vi "VI Tree.vi"   [LabVIEW 2019, in "Agilent 681x Series.lvlib"]
doc: "This is the instrument driver for the Agilent 681x Series. The VI Tree displays all the user-callable VIs of the instrument driver in an organized table."
uses:
  <instrlib>/Agilent 681x Series/Agilent 681x Series.lvlib
  <instrlib>/Agilent 681x Series/Public/Data/Low Level/Fetch Multiple Measurements (Current Data).vi
  <instrlib>/Agilent 681x Series/Public/Data/Read Multiple Measurements (Current Data).vi
  <instrlib>/Agilent 681x Series/Public/Data/Read Single Measurement (Current Harmonics).vi
  <instrlib>/Agilent 681x Series/Public/Data/Low Level/Fetch Single Measurement (Current Harmonics).vi
panel:
  # "(c) 2008-2021 National Instruments Corp.  ALL RIGHTS RESERVED."
  # "SEE DIAGRAM\nFOR VI TREE."
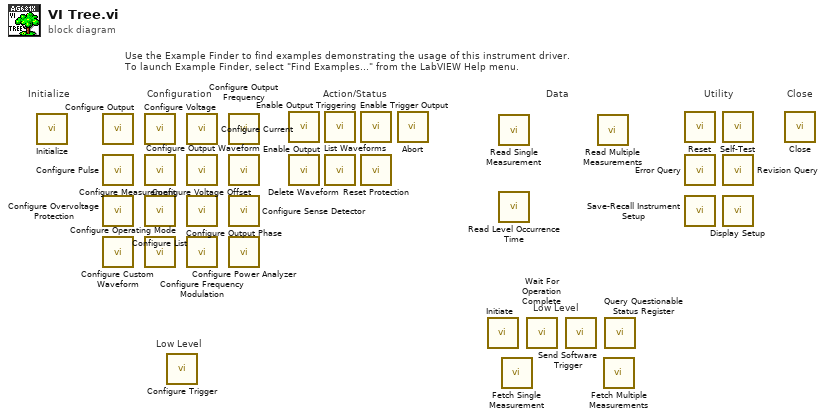
[diagram p0: block diagram]
diagram:
  # "Low Level"
  # "Low Level"
  # "Use the Example Finder to find examples demonstrating the usage of this instrument driver.\nTo launch Example Finder, select \"Find Examples...\" from the LabVIEW Help menu."
  # "Configuration"
  # "Utility"
  # "Data"
  # "Action/Status"
  # "Close"
  # "Initialize"
  n1 = call <instrlib>:"Initialize.vi"() -> ()  [unwired: 10 in, 2 out]
  n2 = call <instrlib>:"Configure Output.vi"() -> ()  [unwired: 14 in, 2 out]
  n3 = call <instrlib>:"Configure Pulse.vi"() -> ()  [unwired: 14 in, 2 out]
  n4 = call <instrlib>:"Configure Overvoltage Protection.vi"() -> ()  [unwired: 14 in, 2 out]
  n5 = call <instrlib>:"Configure Custom Waveform.vi"() -> ()  [unwired: 14 in, 2 out]
  n6 = call <instrlib>:"Configure Voltage.vi"() -> ()  [unwired: 14 in, 2 out]
  n7 = call <instrlib>:"Configure Measurement.vi"() -> ()  [unwired: 14 in, 2 out]
  n8 = call <instrlib>:"Configure List.vi"() -> ()  [unwired: 14 in, 2 out]
  n9 = call <instrlib>:"Configure Operating Mode.vi"() -> ()  [unwired: 14 in, 2 out]
  n10 = call <instrlib>:"Configure Trigger.vi"() -> ()  [unwired: 14 in, 2 out]
  n11 = call <instrlib>:"Configure Current.vi"() -> ()  [unwired: 14 in, 2 out]
  n12 = call <instrlib>:"Configure Voltage Offset.vi"() -> ()  [unwired: 14 in, 2 out]
  n13 = call <instrlib>:"Configure Output Phase.vi"() -> ()  [unwired: 14 in, 2 out]
  n14 = call <instrlib>:"Configure Frequency Modulation.vi"() -> ()  [unwired: 10 in, 2 out]
  n15 = call <instrlib>:"Configure Output Frequency.vi"() -> ()  [unwired: 14 in, 2 out]
  n16 = call <instrlib>:"Configure Output Waveform.vi"() -> ()  [unwired: 14 in, 2 out]
  n17 = call <instrlib>:"Configure Sense Detector.vi"() -> ()  [unwired: 14 in, 2 out]
  n18 = call <instrlib>:"Configure Power Analyzer.vi"() -> ()  [unwired: 10 in, 2 out]
  n19 = call <instrlib>:"Enable Output.vi"() -> ()  [unwired: 14 in, 2 out]
  n20 = call <instrlib>:"Delete Waveform.vi"() -> ()  [unwired: 14 in, 2 out]
  n21 = call <instrlib>:"Enable Output Triggering.vi"() -> ()  [unwired: 14 in, 2 out]
  n22 = call <instrlib>:"List Waveforms.vi"() -> ()  [unwired: 13 in, 3 out]
  n23 = call <instrlib>:"Enable Trigger Output.vi"() -> ()  [unwired: 14 in, 2 out]
  n24 = call <instrlib>:"Reset Protection.vi"() -> ()  [unwired: 14 in, 2 out]
  n25 = call <instrlib>:"Abort.vi"() -> ()  [unwired: 14 in, 2 out]
  n26 = call <instrlib>:"Initiate.vi"() -> ()  [unwired: 10 in, 2 out]
  n27 = call-poly <instrlib>:"Read Single Measurement.vi"() -> ()  [unwired: 10 in, 6 out]
  n28 = call <instrlib>:"Read Level Occurrence Time.vi"() -> ()  [unwired: 8 in, 4 out]
  n29 = call-poly <instrlib>:"Fetch Single Measurement.vi"() -> ()  [unwired: 10 in, 6 out]
  n30 = call <instrlib>:"Wait For Operation Complete.vi"() -> ()  [unwired: 10 in, 2 out]
  n31 = call <instrlib>:"Send Software Trigger.vi"() -> ()  [unwired: 14 in, 2 out]
  n32 = call-poly <instrlib>:"Read Multiple Measurements.vi"() -> ()  [unwired: 11 in, 5 out]
  n33 = call-poly <instrlib>:"Fetch Multiple Measurements.vi"() -> ()  [unwired: 11 in, 5 out]
  n34 = call <instrlib>:"Query Questionable Status Register.vi"() -> ()  [unwired: 9 in, 3 out]
  n35 = call <instrlib>:"Reset.vi"() -> ()  [unwired: 10 in, 2 out]
  n36 = call <instrlib>:"Error Query.vi"() -> ()  [unwired: 8 in, 4 out]
  n37 = call <instrlib>:"Save-Recall Instrument Setup.vi"() -> ()  [unwired: 10 in, 2 out]
  n38 = call <instrlib>:"Self-Test.vi"() -> ()  [unwired: 8 in, 4 out]
  n39 = call <instrlib>:"Revision Query.vi"() -> ()  [unwired: 8 in, 4 out]
  n40 = call <instrlib>:"Display Setup.vi"() -> ()  [unwired: 14 in, 2 out]
  n41 = call <instrlib>:"Close.vi"() -> ()  [unwired: 11 in, 1 out]
